vi "test_libssh2_channel_exec.vi"() -> ()   [LabVIEW 2013, in "libssh2_integration_tests.lvlib"]
uses:
  libssh2_integration_tests.lvlib
  <vilib>/addons/_JKI Toolkits/Caraya/classes/Test/Test.lvclass
  support/support.lvlib
  libssh2/libssh2.lvlib
  <vilib>/addons/_JKI Toolkits/Caraya/classes/Assert/Assert.lvclass
panel:
  out "error out":errorcluster
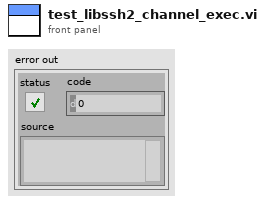
[diagram p1: front panel]
types:
  T1 = typedef "libssh2.lvlib/Session Refnum.ctl" = refnum<k1>
  T2 = typedef "libssh2.lvlib/Channel Refnum.ctl" = refnum<k1>
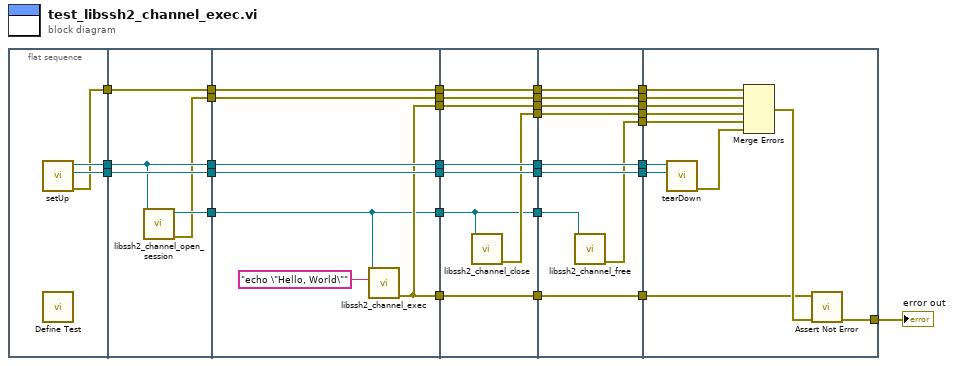
[diagram p0: block diagram]
diagram:
  n1 = flat-sequence {
    tunnel: [w35] -> w32
    tunnel: [w34] -> w31
    tunnel: [w33] -> w30
    tunnel: w32 -> [w39]
    tunnel: w31 -> [w40]
    tunnel: [w39] -> w29
    tunnel: [w40] -> w28
    tunnel: [w38] -> w27
    tunnel: w30 -> [w37]
    tunnel: [w37] -> w26
    tunnel: [w36] -> w25
    tunnel: w29 -> [w47]
    tunnel: [w47] -> w10
    tunnel: w28 -> [w46]
    tunnel: [w46] -> w9
    tunnel: w27 -> [w41]
    tunnel: w26 -> [w45]
    tunnel: [w45] -> w8
    tunnel: w25 -> [w43]
    tunnel: [w43] -> w7
    tunnel: [w42] -> w6
    tunnel: [w42] -> w3
    tunnel: [w41] -> w2
    tunnel: w10 -> [w55]
    tunnel: w9 -> [w54]
    tunnel: [w55] -> w24
    tunnel: [w54] -> w23
    tunnel: [w53] -> w22
    tunnel: w8 -> [w52]
    tunnel: [w52] -> w21
    tunnel: w7 -> [w51]
    tunnel: [w51] -> w20
    tunnel: w6 -> [w50]
    tunnel: [w50] -> w19
    tunnel: [w49] -> w4
    tunnel: w3 -> [w49]
    tunnel: w2 -> [w48]
    tunnel: [w48] -> w1
    tunnel: w24 -> [w64]
    tunnel: w23 -> [w63]
    tunnel: [w64] -> w18
    tunnel: [w63] -> w17
    tunnel: [w62] -> w16
    tunnel: w22 -> [w61]
    tunnel: [w61] -> w15
    tunnel: w21 -> [w60]
    tunnel: [w60] -> w14
    tunnel: w20 -> [w59]
    tunnel: [w59] -> w13
    tunnel: w19 -> [w58]
    tunnel: [w58] -> w12
    tunnel: [w57] -> w5
    tunnel: w4 -> [w57]
    tunnel: w1 -> [w56]
    tunnel: w18 -> [w75]
    tunnel: w17 -> [w74]
    tunnel: [w73] -> w11
    tunnel: w16 -> [w71]
    tunnel: w15 -> [w70]
    tunnel: w14 -> [w69]
    tunnel: w13 -> [w67]
    tunnel: w12 -> [w66]
    tunnel: w5 -> [w65]
    frame #0 {
      n2 = call "setUp.vi"() -> ("error out"=w33:errorcluster, "connection ID"=w34:refnum<k5>, "session"=w35:T1)  [unwired: 9 in]
      n3 = call <vilib>:"Define Test.vi"() -> ()  [unwired: 10 in, 2 out]
    }
    frame #1 {
      n4 = call "libssh2_channel_open_session.vi"("session"=w39) -> ("error out"=w36:errorcluster, "channel"=w38:T2)  [unwired: 9 in]
    }
    frame #2 {
      n5 = call "libssh2_channel_exec.vi"("command"="echo \"Hello, World\"", "channel"=w41) -> ("error out"=w42:errorcluster)  [unwired: 9 in]
    }
    frame #3 {
      n6 = call "libssh2_channel_close.vi"("channel"=w48) -> ("error out"=w53:errorcluster)  [unwired: 10 in]
    }
    frame #4 {
      n7 = call "libssh2_channel_free.vi"("channel"=w56) -> ("error out"=w62:errorcluster)  [unwired: 10 in]
    }
    frame #5 {
      n8 = call "tearDown.vi"("connection ID"=w74, "session"=w75) -> ("error out"=w72:errorcluster)  [unwired: 9 in]
      n9 = Merge Errors(w69, w67, w66, w70, w71, w72) -> (w68:errorcluster)
      n10 = call <vilib>:"Assert Not Error.vi"("error in (no error)"=w68, "Not Error?"=w65) -> ("error out"=w73:errorcluster)  [unwired: 8 in, 1 out]
    }
  }
  "error out" <- w11
